vi "Write ITX (2D w X&Y).vi"(4 "Commands":string, 6 "Notes":string, 8 "error in":errorcluster, 9 "Wavenames":cluster{"2D":string, "X":string, "Y":string}, 10 "2D, X, Y (Cluster)":T1, 11 "filename":path) -> (0 "error out":errorcluster, 3 "file out":path)   [LabVIEW 2016, in "Data.ITX.lvclass"]
uses:
  Data.ITX.lvclass
panel:
  out "String":string
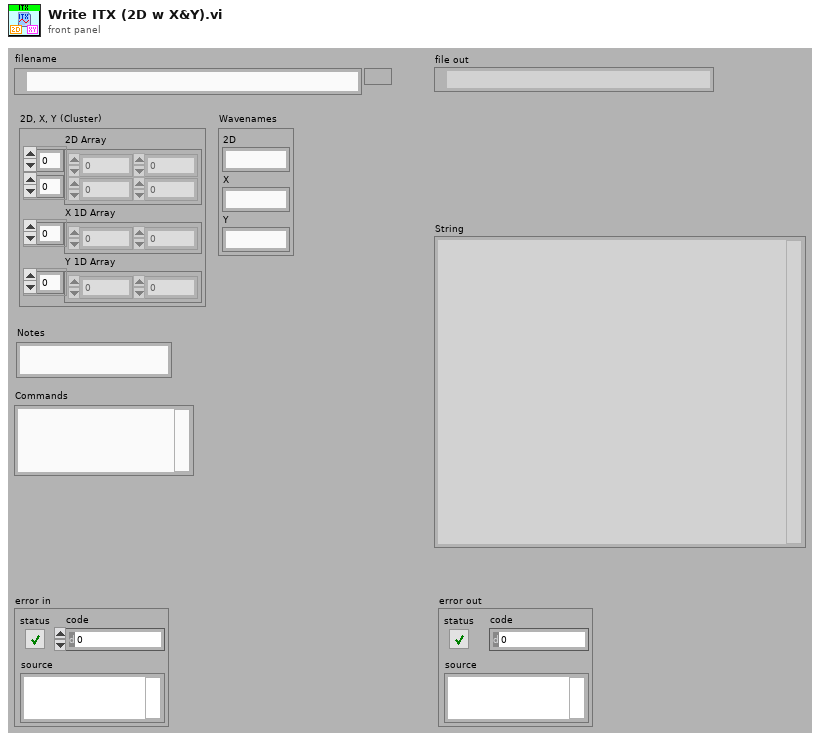
[diagram p1: front panel]
types:
  T1 = cluster{"2D Array":dbl[][], "X 1D Array":dbl[], "Y 1D Array":dbl[]}
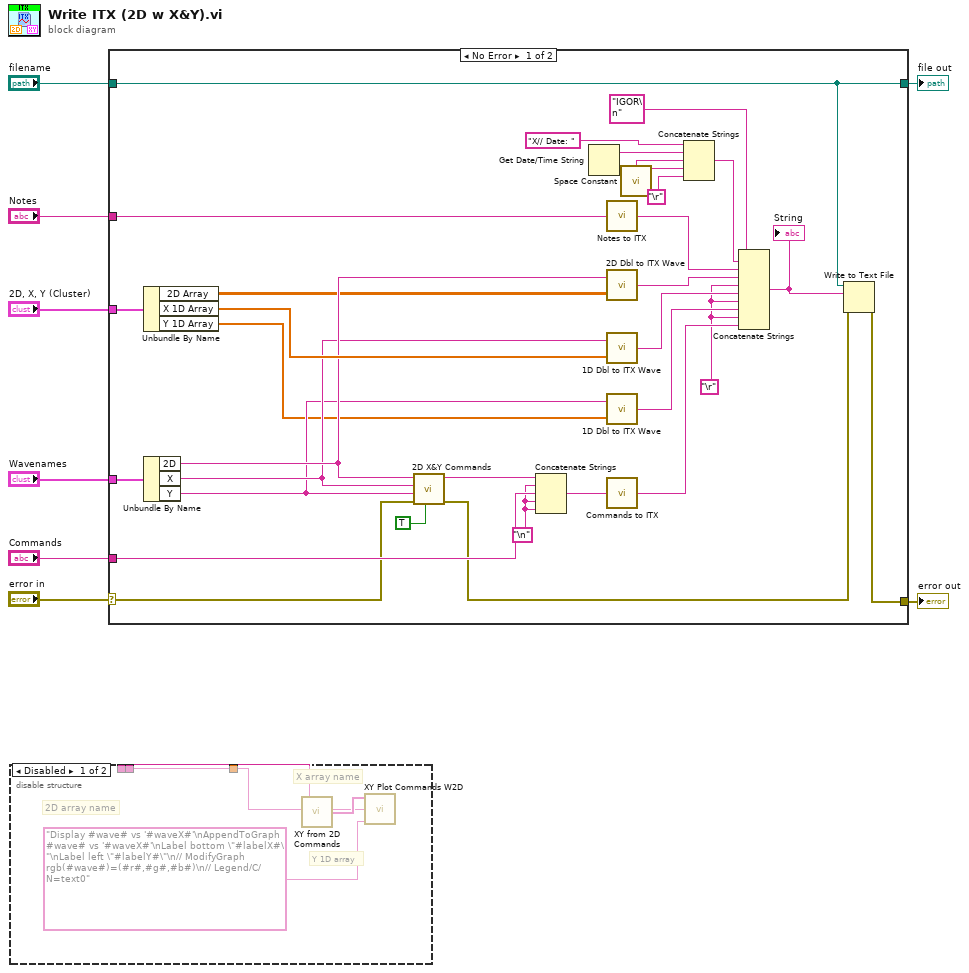
[diagram p0: block diagram]
diagram:
  n1 = disable-structure shown="Disabled" {
    disable-tunnel: _ -> [w13 _]
    disable-tunnel: _ -> [w12 _]
    disable-tunnel: _ -> [w9 _]
    frame Disabled {
      # "Y 1D array"
      # "2D array name"
      # "X array name"
      n2 = call "XY from 2D Commands.vi"("Y 1D Array"=w12, "2D wave"=w13) -> ("wavenames"=w11:string[])
      n3 = call "XY Plot Commands W2D.vi"("wavenames"=w11, "input string"="Display #wave# vs '#waveX#'\nAppendToGraph #wave# vs '#waveX#'\nLabel bottom \"#labelX#\"\nLabel left \"#labelY#\"\n// ModifyGraph rgb(#wave#)=(#r#,#g#,#b#)\n// Legend/C/N=text0", "X wave"=w9) -> ()  [unwired: 2 in, 1 out]
    }
    frame Enabled {
    }
  }
  n4 = case shown="No Error" "error in" {
    selector: "error in" -> [w15 w47]
    tunnel: "Notes" -> [w40 _]
    tunnel: "filename" -> [w24 w46]
    tunnel: "Commands" -> [w28 _]
    tunnel: [w25 w47] -> w4
    tunnel: [w24 w46] -> w3
    tunnel: "2D, X, Y (Cluster)" -> [w23 _]
    tunnel: "Wavenames" -> [w21 _]
    frame No Error {
      w27 = "\n"
      w34 = "\r"
      n5 = Unbundle By Name(w23) -> ("2D Array"=w16:dbl[][], "X 1D Array"=w22:dbl[], "Y 1D Array"=w17:dbl[])
      n6 = Unbundle By Name(w21) -> ("2D"=w20:string, "X"=w19:string, "Y"=w18:string)
      n7 = call "2D X&Y Commands.vi"("Kill X&Y waves?"=TRUE, "error in (no error)"=w15, "Y wave"=w18, "X wave"=w19, "2D wave"=w20) -> ("error out"=w14:errorcluster, "result string"=w29:string)  [unwired: 5 in]
      n8 = Concatenate Strings(w29, w27, w28, w27, w27) -> (w30:string)
      n9 = Get Date/Time String() -> (date string=w44:string, time string=w45:string)  [unwired: 3 out]
      n10 = call "Notes to ITX.vi"("Notes"=w40) -> ("ITX Notes"=w35:string)
      n11 = call "2D Dbl to ITX Wave.vi"("2D Array"=w16, "Wavename"=w20) -> ("ITX Wave"=w39:string)
      n12 = call "1D Dbl to ITX Wave.vi"("1D Array"=w22, "Wavename"=w19) -> ("ITX Wave"=w38:string)
      n13 = call "1D Dbl to ITX Wave.vi"("1D Array"=w17, "Wavename"=w18) -> ("ITX Wave"=w37:string)
      n14 = call "Commands to ITX.vi"("Commands"=w30) -> ("ITX Commands"=w36:string)
      n15 = call <vilib>:"Space Constant.vi"() -> ("String"=w32:string)
      n16 = Concatenate Strings("X// Date: " ("format string"), w44, w32, w45, "\r") -> (w43:string)
      n17 = Concatenate Strings("IGOR\n", w43, w35, w39, w34, w38, w34, w37, w34, w36) -> (w33:string)
      "String" <- w33
      n18 = Write to Text File(file (use dialog)=w24, text=w33, error in=w14) -> (error out=w25:errorcluster)  [unwired: 3 out]
    }
    frame Error {
    }
  }
  "file out" <- w3
  "error out" <- w4
